vi "Fetch Limit Test Result.vi"(8 "error in (no error)":errorcluster, 10 "Limit Line Number (1: Line 1)":i32(ring)=1 items=["Line1"=1, "Line2"=2], 11 "VISA resource name":refnum<visa-resource-name>) -> (0 "error out":errorcluster, 2 "Limit Test Result":dbl, 3 "VISA resource name out":refnum<visa-resource-name>)   [LabVIEW 2022 SP3, in "Agilent N934X Series.lvlib"]
doc: "Fetch the limits pass/failed result.\n\nNote:\n\nThis VI does not check the instrument status. Typically, you call this VI only in a sequence of calls to other low-level instrument driver VIs. The sequence performs one operation. You use the low-level VIs to optimize one or more aspects of interaction with the instrument. If you want to check the instrument status, call the <B>Error Query VI</B> at the conclusion of the sequence."
uses:
  <instrlib>/Agilent N934X Series/Agilent N934X Series.lvlib
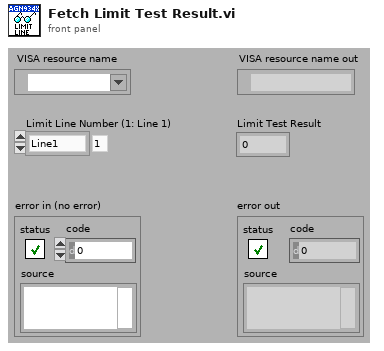
[diagram p1: front panel]
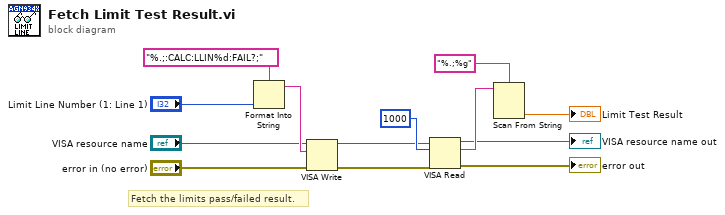
[diagram p0: block diagram]
diagram:
  # "Fetch the limits pass/failed result."
  n1 = Format Into String(format string="%.;:CALC:LLIN%d:FAIL?;", "Limit Line Number (1: Line 1)") -> (resulting string=w11:string)  [unwired: 2 in, 1 out]
  n2 = VISA Write(VISA resource name="VISA resource name", write buffer=w11, error in (no error)="error in (no error)") -> (VISA resource name out=w5:refnum<visa-resource-name>, error out=w4:errorcluster)  [unwired: 1 out]
  n3 = VISA Read(VISA resource name=w5, byte count=u32 1000, error in (no error)=w4) -> (VISA resource name out=→"VISA resource name out":refnum<visa-resource-name>, read buffer=w6:string, error out=→"error out":errorcluster)  [unwired: 1 out]
  n4 = Scan From String(format string="%.;%g", input string=w6) -> (output 1=→"Limit Test Result":dbl)  [unwired: 3 in, 3 out]
